vi "ObtainQueue_Shell.vi"(8 "error in (no error)":errorcluster) -> (0 "error out":errorcluster, 3 "queue out":refnum<queue>)   [LabVIEW 2019]
uses:
  LvProviderShellHelper/LvProviderShellHelper.lvclass
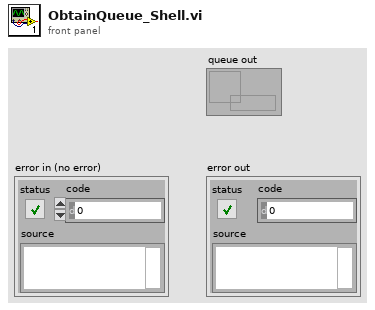
[diagram p1: front panel]
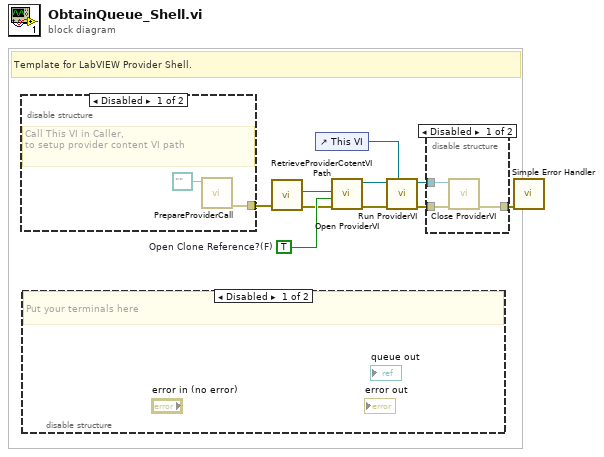
[diagram p0: block diagram]
diagram:
  w6 = TRUE  # Open Clone Reference?(F)
  # "Template for LabVIEW Provider Shell."
  n1 = disable-structure shown="Disabled" {
    disable-tunnel: [w12 _] -> w1
    frame Disabled {
      # "Call This VI in Caller, \nto setup provider content VI path"
      n2 = call "PrepareProviderCall.vi"("ProviderCotentVI Path"=path "") -> ("error out"=w12:errorcluster)  [unwired: 10 in]
    }
    frame Enabled {
    }
  }
  n3 = disable-structure shown="Disabled" {
    frame Disabled {
      # "Put your terminals here"
    }
    frame Enabled {
    }
  }
  n4 = call "RetrieveProviderCotentVIPath.vi"("error in (no error)"=w1) -> ("error out"=w3:errorcluster, "Initialize-API"=w2:path)  [unwired: 9 in]
  n5 = control-ref of="This VI"() -> (w5:refnum<vi>)
  n6 = call "Open ProviderVI.vi"("error in (no error)"=w3, "Open Clone Reference?(F)"=w6, "vi path"=w2) -> ("error out"=w8:errorcluster, "vi reference"=w4:refnum<vi>)  [unwired: 7 in]
  n7 = call "Run ProviderVI.vi"("Shell VI"=w5, "error in (no error)"=w8, "vi reference"=w4) -> ("error out"=w9:errorcluster, "VI out"=w10:refnum<vi>)  [unwired: 7 in]
  n8 = disable-structure shown="Disabled" {
    disable-tunnel: w10 -> [w15 _]
    disable-tunnel: w9 -> [w14 w16]
    disable-tunnel: [w13 w16] -> w7
    frame Disabled {
      n9 = call "Close ProviderVI.vi"("error in (no error)"=w14, "VI in"=w15) -> ("error out"=w13:errorcluster)  [unwired: 9 in]
    }
    frame Enabled {
    }
  }
  n10 = call <vilib>:"Simple Error Handler.vi"("error in (no error)"=w7) -> ()  [unwired: 4 in, 5 out]
